vi "Sequence.Test.UpdateCounters.vi"(8 "error in":errorcluster, 10 "Status.Prod":T1[](array[typedef]), 11 "Code in":T7={"Ready"=FALSE, "DoubleOrder"=FALSE, "OrderDone"=FALSE, "AllowSingleSlot"=FALSE, "CheckDM"=FALSE, "ThresholdA"=0, "ThresholdB"=0, "Plate"=enum."Wabco", "ImgPath"=path "", "Variant"={"State"=enum."Init", "ImgPath"=path "", "WabcoPlate"="", "WabcoProduct"="", "ClientProduct"="", "ClientPlate"="", "TotalQuantity"=0, "OrderQuantity"=0, "Serial"=0, "Wabco"={"LaserJob"="", "AdditionalTxt"="037", "FactoryCode"="", "RevID"=0, "ForkID"=0, "FailuresLimit"=0, "GlobalCnt"=0, "ScannerProgram"=0, "SerialFormat"=enum."6 dig", "CoordA"={"X"=0.0, "Y"=0.0, "Angle"=0.0}, "CoordB"={"X"=0.0, "Y"=0.0, "Angle"=0.0}, "DMCconfig"=0}, "Client"={"LaserJob"="", "AdditionalTxt"="", "FactoryCode"="037", "RevID"=0, "ForkID"=0, "FailuresLimit"=0, "GlobalCnt"=0, "ScannerProgram"=0, "SerialFormat"=enum."6 dig", "CoordA"={"X"=0.0, "Y"=0.0, "Angle"=0.0}, "CoordB"={"X"=0.0, "Y"=0.0, "Angle"=0.0}, "DMCconfig"=0}}}) -> (0 "error out":errorcluster, 2 "Printed serials out":i32[](array[numeric]), 3 "Code out":T7={"Ready"=FALSE, "DoubleOrder"=FALSE, "OrderDone"=FALSE, "AllowSingleSlot"=FALSE, "CheckDM"=FALSE, "ThresholdA"=0, "ThresholdB"=0, "Plate"=enum."Wabco", "ImgPath"=path "", "Variant"={"State"=enum."Init", "ImgPath"=path "", "WabcoPlate"="", "WabcoProduct"="", "ClientProduct"="", "ClientPlate"="", "TotalQuantity"=0, "OrderQuantity"=0, "Serial"=0, "Wabco"={"LaserJob"="", "AdditionalTxt"="037", "FactoryCode"="", "RevID"=0, "ForkID"=0, "FailuresLimit"=0, "GlobalCnt"=0, "ScannerProgram"=0, "SerialFormat"=enum."6 dig", "CoordA"={"X"=0.0, "Y"=0.0, "Angle"=0.0}, "CoordB"={"X"=0.0, "Y"=0.0, "Angle"=0.0}, "DMCconfig"=0}, "Client"={"LaserJob"="", "AdditionalTxt"="", "FactoryCode"="037", "RevID"=0, "ForkID"=0, "FailuresLimit"=0, "GlobalCnt"=0, "ScannerProgram"=0, "SerialFormat"=enum."6 dig", "CoordA"={"X"=0.0, "Y"=0.0, "Angle"=0.0}, "CoordB"={"X"=0.0, "Y"=0.0, "Angle"=0.0}, "DMCconfig"=0}}})   [LabVIEW 2016]
uses:
  Global/ApplicationGlobal.vi
  Station/Station.Changeover.State.vi
  Sequence.Code.SerialFormat.ctl
  Drivers/V7310/LowLevel/V7310.Job.Sets.ctl
  Station/Station.Plate.Properties.ctl
  Logger/Logger.Variant.Sets.ctl
  Sequence.Code.Sets.ctl
  Sequence.PlateType.ctl
  Sequence.Step.Status.ctl
  Sequence.Test.BreakReason.ctl
  Sequence.Prod.StatusData.ctl
  Sequence.Test.Unload.Status.ctl
  Sequence.Slot.StatusData.ctl
  Sequence.Test.Status.ctl
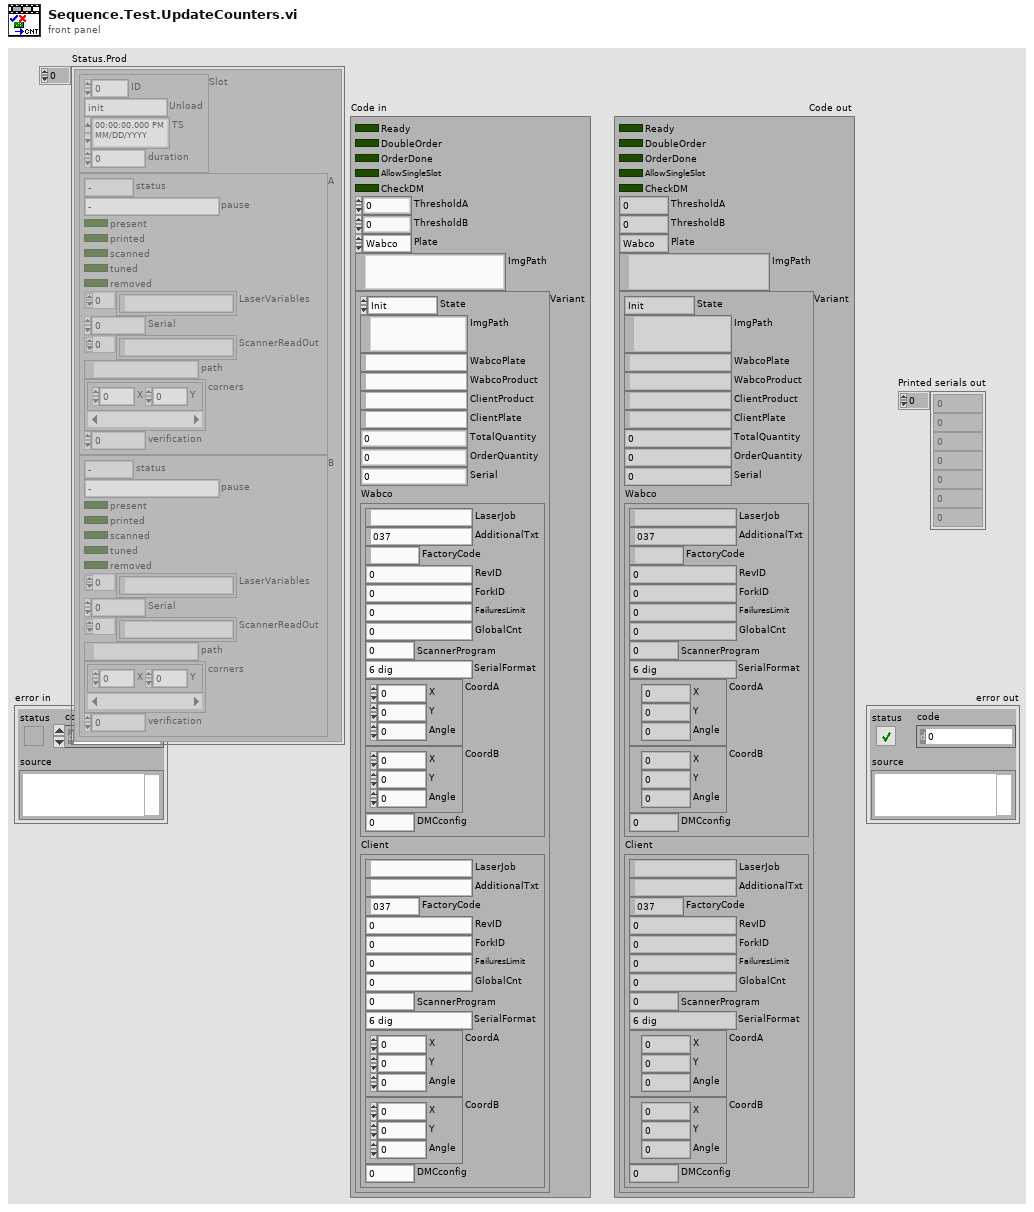
[diagram p1: front panel]
types:
  T1 = typedef "Sequence.Test.Status.ctl" = cluster{"Slot":T2, "A":T4, "B":T4}
  T2 = typedef "Sequence.Slot.StatusData.ctl" = cluster{"ID":i32, "Unload":T3, "TS":timestamp, "duration":u32}
  T3 = typedef "Sequence.Test.Unload.Status.ctl" = enum16{"init", "check NOK", "check OK", "wait on NOK", "wait on OK", "wait on Unload", "done"}
  T4 = typedef "Sequence.Prod.StatusData.ctl" = cluster{"status":T5, "pause":T6, "present":bool, "printed":bool, "scanned":bool, "tuned":bool, "removed":bool, "LaserVariables":string[], "Serial":i32, "ScannerReadOut":string[], "path":path, "corners":cluster{"X":i32, "Y":i32}[], "verification":u8}
  T5 = typedef "Sequence.Step.Status.ctl" = enum16{"-", "Pending", "Running", "Skipped", "Passed", "Failed", "Done", "Error", "Aborted", "Stopped"}
  T6 = typedef "Sequence.Test.BreakReason.ctl" = enum16{"-", "NOK container", "OK container", "Rev empty", "Rev missing", "Rev wrong", "Fork missing", "Fork wrong", "NOK limit", "Unload failure", "Single slot", "Part done", "Err: Prod move work", "Err: Prod move home", "Err: Prod lift work", "Err: Prod lift home", "Err: Prod Arm Work", "Err: Prod Arm NOK", "Err: Prod Arm OK", "Err: Prod NOK suck", "Err: Prod NOK drop", "Err: Prod OK missing", "Err: Prod OK suck", "Err: Prod OK drop"}
  T7 = typedef "Sequence.Code.Sets.ctl" = cluster{"Ready":bool, "DoubleOrder":bool, "OrderDone":bool, "AllowSingleSlot":bool, "CheckDM":bool, "ThresholdA":u8, "ThresholdB":u8, "Plate":T8, "ImgPath":path, "Variant":T9}
  T8 = typedef "Sequence.PlateType.ctl" = enum16{"Wabco", "Client"}
  T9 = typedef "Logger.Variant.Sets.ctl" = cluster{"State":T10, "ImgPath":path, "WabcoPlate":string, "WabcoProduct":string, "ClientProduct":string, "ClientPlate":string, "TotalQuantity":u16, "OrderQuantity":u16, "Serial":i32, "Wabco":T11, "Client":T11}
  T10 = typedef "Station.Changeover.State.vi" = enum16{"Init", "Scaning", "NOK", "Wait for ack", "Ready"}
  T11 = typedef "Station.Plate.Properties.ctl" = cluster{"LaserJob":string, "AdditionalTxt":string, "FactoryCode":string, "RevID":u8, "ForkID":u8, "FailuresLimit":u16, "GlobalCnt":i32, "ScannerProgram":u8, "SerialFormat":T12, "CoordA":T13, "CoordB":T13, "DMCconfig":i32}
  T12 = typedef "Sequence.Code.SerialFormat.ctl" = enum8{"", "6 dig", "7 dig"}
  T13 = typedef "V7310.Job.Sets.ctl" = cluster{"X":dbl, "Y":dbl, "Angle":dbl}
  T14 = typedef "Sequence.SerialsFglb.StatusFlags.ctl" = cluster{"Global":bool, "NokLimit":bool, "PartDone":bool, "Completed":bool}
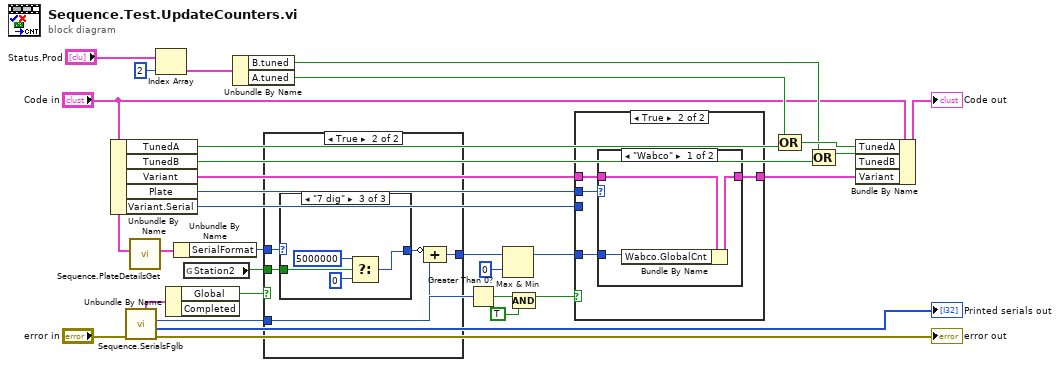
[diagram p0: block diagram]
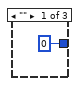
[diagram p3: hidden frame]
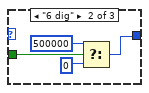
[diagram p4: hidden frame]
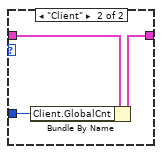
[diagram p6: hidden frame]
diagram:
  n1 = Unbundle By Name("Code in") -> ("TunedA"=w19:bool, "TunedB"=w16:bool, "Variant"=w27:T9, "Plate"=w28:T8, "Variant.Serial"=w26:i32)
  n2 = call "Sequence.SerialsFglb.vi"("error in"="error in") -> ("error out"=→"error out":errorcluster, "Printed serials out"=→"Printed serials out":i32[], "Serial out"=w9:i32, "StatusFlags"=w5:T14)  [unwired: 6 in, 1 out]
  n3 = call "Sequence.PlateDetailsGet.vi"("Code in"="Code in") -> ("PlateDetails"=w11:T11)  [unwired: 9 in, 1 out]
  n4 = Index Array(array="Status.Prod", index=2) -> (element=w20:T1)
  n5 = Unbundle By Name(w5) -> ("Global"=w4:bool)  [unwired: 1 out]
  n6 = Unbundle By Name(w11) -> ("SerialFormat"=w12:T12)
  n7 = global read "ApplicationGlobal.vi" "Station2"() -> (w3:bool)
  n8 = Unbundle By Name(w20) -> ("B.tuned"=w14:bool, "A.tuned"=w18:bool)
  n9 = case shown="True" w4 {
    tunnel: w12 -> [_ w36]
    tunnel: w9 -> [w31 w34]
    tunnel: [w31 w33] -> w7
    tunnel: w3 -> [_ w32]
    frame False {
    }
    frame True {
      n10 = case shown="\"7 dig\"" w36 {
        tunnel: [0 ("Serial") w38 w42] -> w35
        tunnel: w32 -> [_ w41 w43]
        frame "" {
        }
        frame "6 dig" {
          n11 = Select(t=500000 ("Serial"), s=w41, f=0 ("Serial")) -> (s? t:f=w38:i32)
        }
        frame "7 dig" {
          n12 = Select(t=5000000 ("Serial"), s=w43, f=0 ("Serial")) -> (s? t:f=w42:i32)
        }
      }
      n13 = Compound Arithmetic op=ADD(invert w35, w34) -> (w33:i32)
    }
  }
  n14 = Greater Than 0?(x=w9) -> (x > 0?=w8:bool)
  n15 = Max & Min(x=w7, y=0 ("x")) -> (max(x,y)=w10:i32)  [unwired: 1 out]
  n16 = Compound Arithmetic op=AND(w8, TRUE) -> (w2:bool)
  n17 = case shown="True" w2 {
    tunnel: w28 -> [_ w50]
    tunnel: w27 -> [w46 w49]
    tunnel: w26 -> [_ _]
    tunnel: [w46 w48] -> w25
    tunnel: w10 -> [_ w47]
    frame False {
    }
    frame True {
      n18 = case shown="\"Wabco\"" w50 {
        tunnel: w49 -> [w53 w56]
        tunnel: w47 -> [w52 w55]
        tunnel: [w51 w54] -> w48
        frame "Wabco" {
          n19 = Bundle By Name(cluster=w53, "Wabco.GlobalCnt"=w52) -> (w51:T9)
        }
        frame "Client" {
          n20 = Bundle By Name(cluster=w56, "Client.GlobalCnt"=w55) -> (w54:T9)
        }
      }
    }
  }
  n21 = Compound Arithmetic op=OR(w18, w19) -> (w17:bool)
  n22 = Compound Arithmetic op=OR(w14, w16) -> (w15:bool)
  n23 = Bundle By Name(cluster="Code in", "TunedA"=w17, "TunedB"=w15, "Variant"=w25) -> (→"Code out":T7)
